vi "RainbowStationMain.vi"(8 "error in (no error)":errorcluster) -> (0 "error out":errorcluster={"status"=FALSE, "code"=1073676418, "source"="VISA Close in RainbowStationMain.vi"})   [LabVIEW 2013]
doc: "Use this template to build a VI to use as a subVI."
uses:
  GRIMM/GRIMMstatusEnum.ctl
  GRIMM/GRIMMmeasurementEnum.ctl
  HighVolumeSampler/HVSmeasurementEnum.ctl
  <vilib>/Instr/_visa.llb/Select Event Type.ctl
  Nephelometer/NephDataEnum.ctl
  GRIMM/GRIMMErrorMessage.ctl
  GRIMM/GRIMMmeasurementCluster.ctl
  <vilib>/Instr/_visa.llb/VISA Configure Serial Port (Instr).vi
  <vilib>/Utility/file.llb/Write To Spreadsheet File (string).vi
  HighVolumeSampler/X-Modem_Labview85/Xmodem VISA.llb/XMODEM Type.ctl
panel:
  out "Pressure (mbar)":dbl(slide)=1007.3810320000001 scale=1000.0..1020.0
  out "Wind Direction":i32(knob)=170 scale=0.0..359.0
  out "Wind Speed":dbl(knob)=0.014 scale=0.0..28.0
  out "Humidity":dbl(slide)=48.6 scale=0.0..100.0
  out "Temperature":dbl(slide)=20.789 scale=0.0..100.0
  in  "error in (no error) 3":errorcluster
  out "XY Graph":cluster{dbl[], dbl[]}[](graph)=[{[0.25, 0.28], [1170.3030084322447, 1170.3030084322447]}, {[0.28, 0.3], [1293.252048081437, 1293.252048081437]}, {[0.3, 0.35], [433.9267074685252, 433.9267074685252]}, {[0.35, 0.4], [288.83320655615836, 288.83320655615836]}, {[0.4, 0.45], [74.28763662454614, 74.28763662454614]}, {[0.45, 0.5], [40.43053885454822, 40.43053885454822]}, {[0.5, 0.58], [42.66344688970791, 42.66344688970791]}, {[0.58, 0.65], [14.145596928722288, 14.145596928722288]}, {[0.65, 0.7], [21.74947604493162, 21.74947604493162]}, {[0.7, 0.8], [14.65720749687968, 14.65720749687968]}, {[0.8, 1.0], [8.255080926812933, 8.255080926812933]}, {[1.0, 1.3], [2.632887254292233, 2.632887254292233]}, {[1.3, 1.6], [2.2178695214687925, 2.2178695214687925]}, {[1.6, 2.0], [3.09565534755485, 3.09565534755485]}, {[2.0, 2.5], [2.373335766458719, 2.373335766458719]}, {[2.5, 3.0], [1.010340250921067, 1.010340250921067]}, {[3.0, 3.5], [1.1949788845949056, 1.1949788845949056]}, {[3.5, 4.0], [0.8621886762870412, 0.8621886762870412]}, {[4.0, 5.0], [0.9286966042664552, 0.9286966042664552]}, {[5.0, 6.5], [0.08776290847640775, 0.08776290847640775]}, {[6.5, 7.5], [0.0, 0.0]}, {[7.5, 8.5], [0.0, 0.0]}, {[8.5, 10.0], [0.0, 0.0]}, {[10.0, 12.5], [0.1031885115851617, 0.1031885115851617]}, {[12.5, 15.0], [0.0, 0.0]}, {[15.0, 17.5], [0.0, 0.0]}, {[17.5, 20.0], [0.0, 0.0]}, {[20.0, 25.0], [0.0, 0.0]}, {[25.0, 30.0], [0.0, 0.0]}, {[30.0, 32.0], [0.0, 0.0]}]
  out "Number of Particles":i32[](array[numeric])=[15495, 9735, 5860, 2955, 1280, 900, 715, 440, 370, 300, 215, 135, 105, 85, 55, 32, 32, 24, 16, 11, 2, 1, 1, 1, 1, 0, 0, 0, 0, 0, 0, 0]
  in  "error in (no error) 2":errorcluster
  in  "Save HVS file":bool
  in  "HVS File Path":path
  in  "HVS Com Port":refnum<visa-resource-name>="COM1"
  in  "Simulation Mode":bool
  in  "Set Interval Time Button":bool
  in  "Interval Time":T1(ring)=enum."6 Seconds"
  in  "Stop GRIMM Measurement":bool
  in  "Start GRIMM Measurement":bool
  in  "stop":bool
  in  "Save GRIMM file":bool
  in  "GRIMM File Path":path
  in  "GRIMM Com Port":refnum<visa-resource-name>="COM2"
  in  "Save Neph File":bool
  in  "File Path Control":path=path "T:/LabBox/Software/Airphoton Nephelometer/TestMean.csv"
  in  "Nephelometer Com Port":refnum<visa-resource-name>="COM17"
  out "Total Scattering (Red (632nm), Green (532nm), Blue (450nm))":waveform(dbl)[](graph)=[{"t0"=timestamp(3528791463.22 s since 1904-01-01), "dt"=1.0, "Y"=[11.768620561478]}, {"t0"=timestamp(3528791463.22 s since 1904-01-01), "dt"=1.0, "Y"=[10.3616270811]}, {"t0"=timestamp(3528791463.22 s since 1904-01-01), "dt"=1.0, "Y"=[32.318224076812]}]
  out "External Sensors":waveform(dbl)[](graph)=[{"t0"=timestamp(3528791463.22 s since 1904-01-01), "dt"=1.0, "Y"=[24.22]}, {"t0"=timestamp(3528791463.22 s since 1904-01-01), "dt"=1.0, "Y"=[101.15]}, {"t0"=timestamp(3528791463.22 s since 1904-01-01), "dt"=1.0, "Y"=[48.6]}]
  out "Counts vs Time":waveform(dbl)[](graph)=[{"t0"=timestamp(3528791463.266 s since 1904-01-01), "dt"=1.0, "Y"=[154.95000000000002]}, {"t0"=timestamp(3528791463.266 s since 1904-01-01), "dt"=1.0, "Y"=[153.60000000000002]}, {"t0"=timestamp(3528791463.266 s since 1904-01-01), "dt"=1.0, "Y"=[154.63000000000002]}, {"t0"=timestamp(3528791463.266 s since 1904-01-01), "dt"=1.0, "Y"=[154.94000000000003]}]
  out "Meterological Data":waveform(dbl)[](graph)=[{"t0"=timestamp(3528791462.555 s since 1904-01-01), "dt"=1.0, "Y"=[755.6]}, {"t0"=timestamp(3528791462.555 s since 1904-01-01), "dt"=1.0, "Y"=[20.789]}]
  out "Meterological Data 2":waveform(dbl)[](graph)=[{"t0"=timestamp(3528791462.555 s since 1904-01-01), "dt"=1.0, "Y"=[0.014]}, {"t0"=timestamp(3528791462.555 s since 1904-01-01), "dt"=1.0, "Y"=[169.94]}]
  out "High Volume Sampler - Sampling Data":waveform(dbl)[](graph)=[{"t0"=timestamp(3528791462.555 s since 1904-01-01), "dt"=1.0, "Y"=[0.0]}, {"t0"=timestamp(3528791462.555 s since 1904-01-01), "dt"=1.0, "Y"=[0.0]}, {"t0"=timestamp(3528791462.555 s since 1904-01-01), "dt"=1.0, "Y"=[0.0]}]
  out "XY Graph 2":cluster{dbl[], dbl[]}[](graph)=[{[0.25, 0.28], [57.60000000000001, 57.60000000000001]}, {[0.28, 0.3], [38.75000000000001, 38.75000000000001]}, {[0.3, 0.35], [29.05, 29.05]}, {[0.35, 0.4], [16.75, 16.75]}, {[0.4, 0.45], [3.8000000000000007, 3.8000000000000007]}, {[0.45, 0.5], [1.8499999999999996, 1.8499999999999996]}, {[0.5, 0.58], [2.75, 2.75]}, {[0.58, 0.65], [0.7000000000000002, 0.7000000000000002]}, {[0.65, 0.7], [0.7000000000000002, 0.7000000000000002]}, {[0.7, 0.8], [0.8500000000000001, 0.8500000000000001]}, {[0.8, 1.0], [0.7999999999999998, 0.7999999999999998]}, {[1.0, 1.3], [0.30000000000000004, 0.30000000000000004]}, {[1.3, 1.6], [0.20000000000000007, 0.20000000000000007]}, {[1.6, 2.0], [0.29999999999999993, 0.29999999999999993]}, {[2.0, 2.5], [0.23000000000000004, 0.23000000000000004]}, {[2.5, 3.0], [0.08000000000000002, 0.08000000000000002]}, {[3.0, 3.5], [0.07999999999999999, 0.07999999999999999]}, {[3.5, 4.0], [0.05, 0.05]}, {[4.0, 5.0], [0.09, 0.09]}, {[5.0, 6.5], [0.01, 0.01]}, {[6.5, 7.5], [0.0, 0.0]}, {[7.5, 8.5], [0.0, 0.0]}, {[8.5, 10.0], [0.0, 0.0]}, {[10.0, 12.5], [0.01, 0.01]}, {[12.5, 15.0], [0.0, 0.0]}, {[15.0, 17.5], [0.0, 0.0]}, {[17.5, 20.0], [0.0, 0.0]}, {[20.0, 25.0], [0.0, 0.0]}, {[25.0, 30.0], [0.0, 0.0]}, {[30.0, 32.0], [0.0, 0.0]}]
  out "Battery Power (%)":i32
  out "Power Supply Type":T2(ring)
  out "Pump Current (%)":i32 format="Pump Current %.0f %%"
  out "Error Messages":u16(ring) items=["New SELF-TEST: Fault Self-Test"=128, "No Memory Card"=64, "Check Nozzle: Whirls > 5%"=32, "No Operation: Battery Capacity = 0%"=16, "Please Recharge: Battery Capacity < 10%"=8, "Pump Current too High - Motor Current Imot > 100%"=4, "Flow-Error: Volume flow control out of control range"=3, "Check Filter Imot < 20% "=2, "Check Filter Imot > 60%"=1, "No Error :)"=0]
  out "read buffer 2":string="1024,9/17/15 10:52:54,3093186,10310875,2353742,4299422,4381491,6981848,1595346,20761660,1351020,7590174,2065561,14187844,24.22,101.15,48.6,874857,984521,1006387,4.775941096085,5.786920205497,5.869425532089,11.768620561478,10.361627081100,32.318224076812,0\u0000"
  out "read buffer":string="C9:   15495     9735     5860     2955     1280      900      715      440 \nC9;     370      300      215      135      105       85       55       32 \nc9:      32       24       16       11        2        1        1        1 \nc9;       1        0        0        0        0        0        0        0 \n"
  in  "error in (no error) 5":errorcluster
  out "HVS RAW data":string
  in  "Array":dbl[](array[numeric])
  out "error out 2":errorcluster
  in  "error in (no error) 4":errorcluster
  # "m/s"
  # "%"
  # "C"
  # "N"
  # "W"
  # "E"
  # "S"
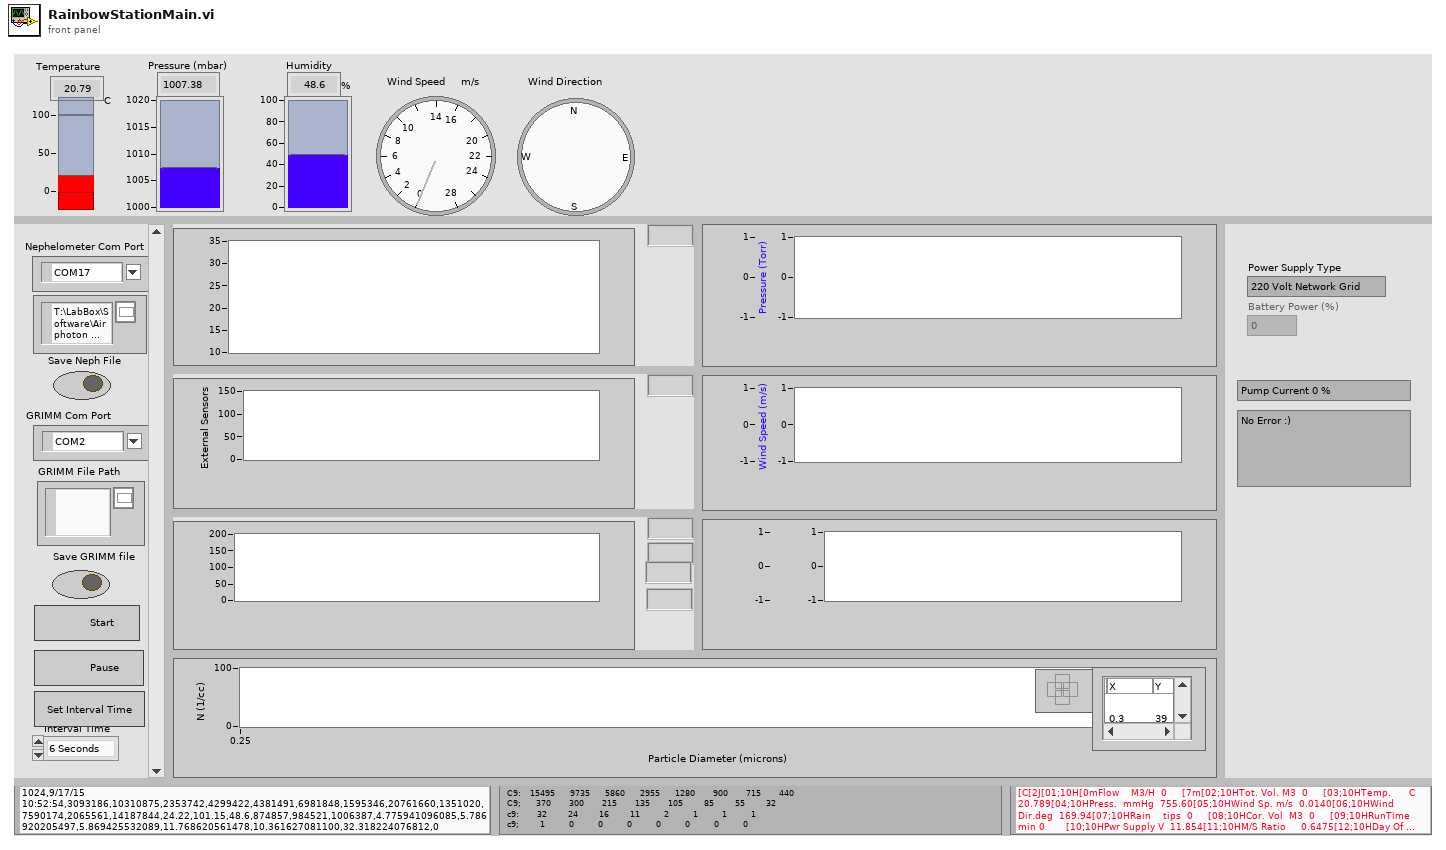
[diagram p1: front panel]
types:
  T1 = enum16{"1 Minute", "5 Mintues", "10 Minutes", "15 Minutes", "30 Minutes", "60 Minutes", "6 Seconds", "3 Seconds", "2 Seconds", "1 Second"}
  T2 = enum16{"220 Volt Network Grid", "Battery Powered"}
  T3 = typedef "NephDataEnum.ctl" = enum16{"Init", "Insert Measurement", "Read Buffer Size", "Write Buffer Size", "Read Current Measurement", "Read All Buffered Meas"}
  T4 = typedef "Select Event Type.ctl" = u32
  T5 = typedef "HVSmeasurementEnum.ctl" = enum16{"Get WindSpeedDirectionVsTime", "Get VolumeFlowrateVsTime", "Get PressureTempVsTime", "InsertMeasurement", "Init"}
  T6 = typedef "GRIMMmeasurementEnum.ctl" = enum16{"Save Raw to file", "Get NvsDiameter", "Get DNDlogDPVsDiameter", "Get CountsVsTime", "Get Raw Data", "InsertMeasurement", "Init"}
  T7 = typedef "GRIMMstatusEnum.ctl" = enum16{"Get Pump Current", "Get Power Supply Type", "Get Battery Power", "Get Error message", "Get Instrument DateTime", "Insert Status Data", "Init"}
  T8 = typedef "GRIMMmeasurementCluster.ctl" = cluster{"Threshold Bin size":dbl[], "Measurement Data":i32[]}
  T9 = enum8{"Enabled", "Disabled", "Disabled and Grayed Out"}
  T10 = typedef "GRIMMErrorMessage.ctl" = u16
  T11 = typedef "XMODEM Type.ctl" = enum16{"XMODEM", "XMODEM-CRC", "XMODEM-1K"}
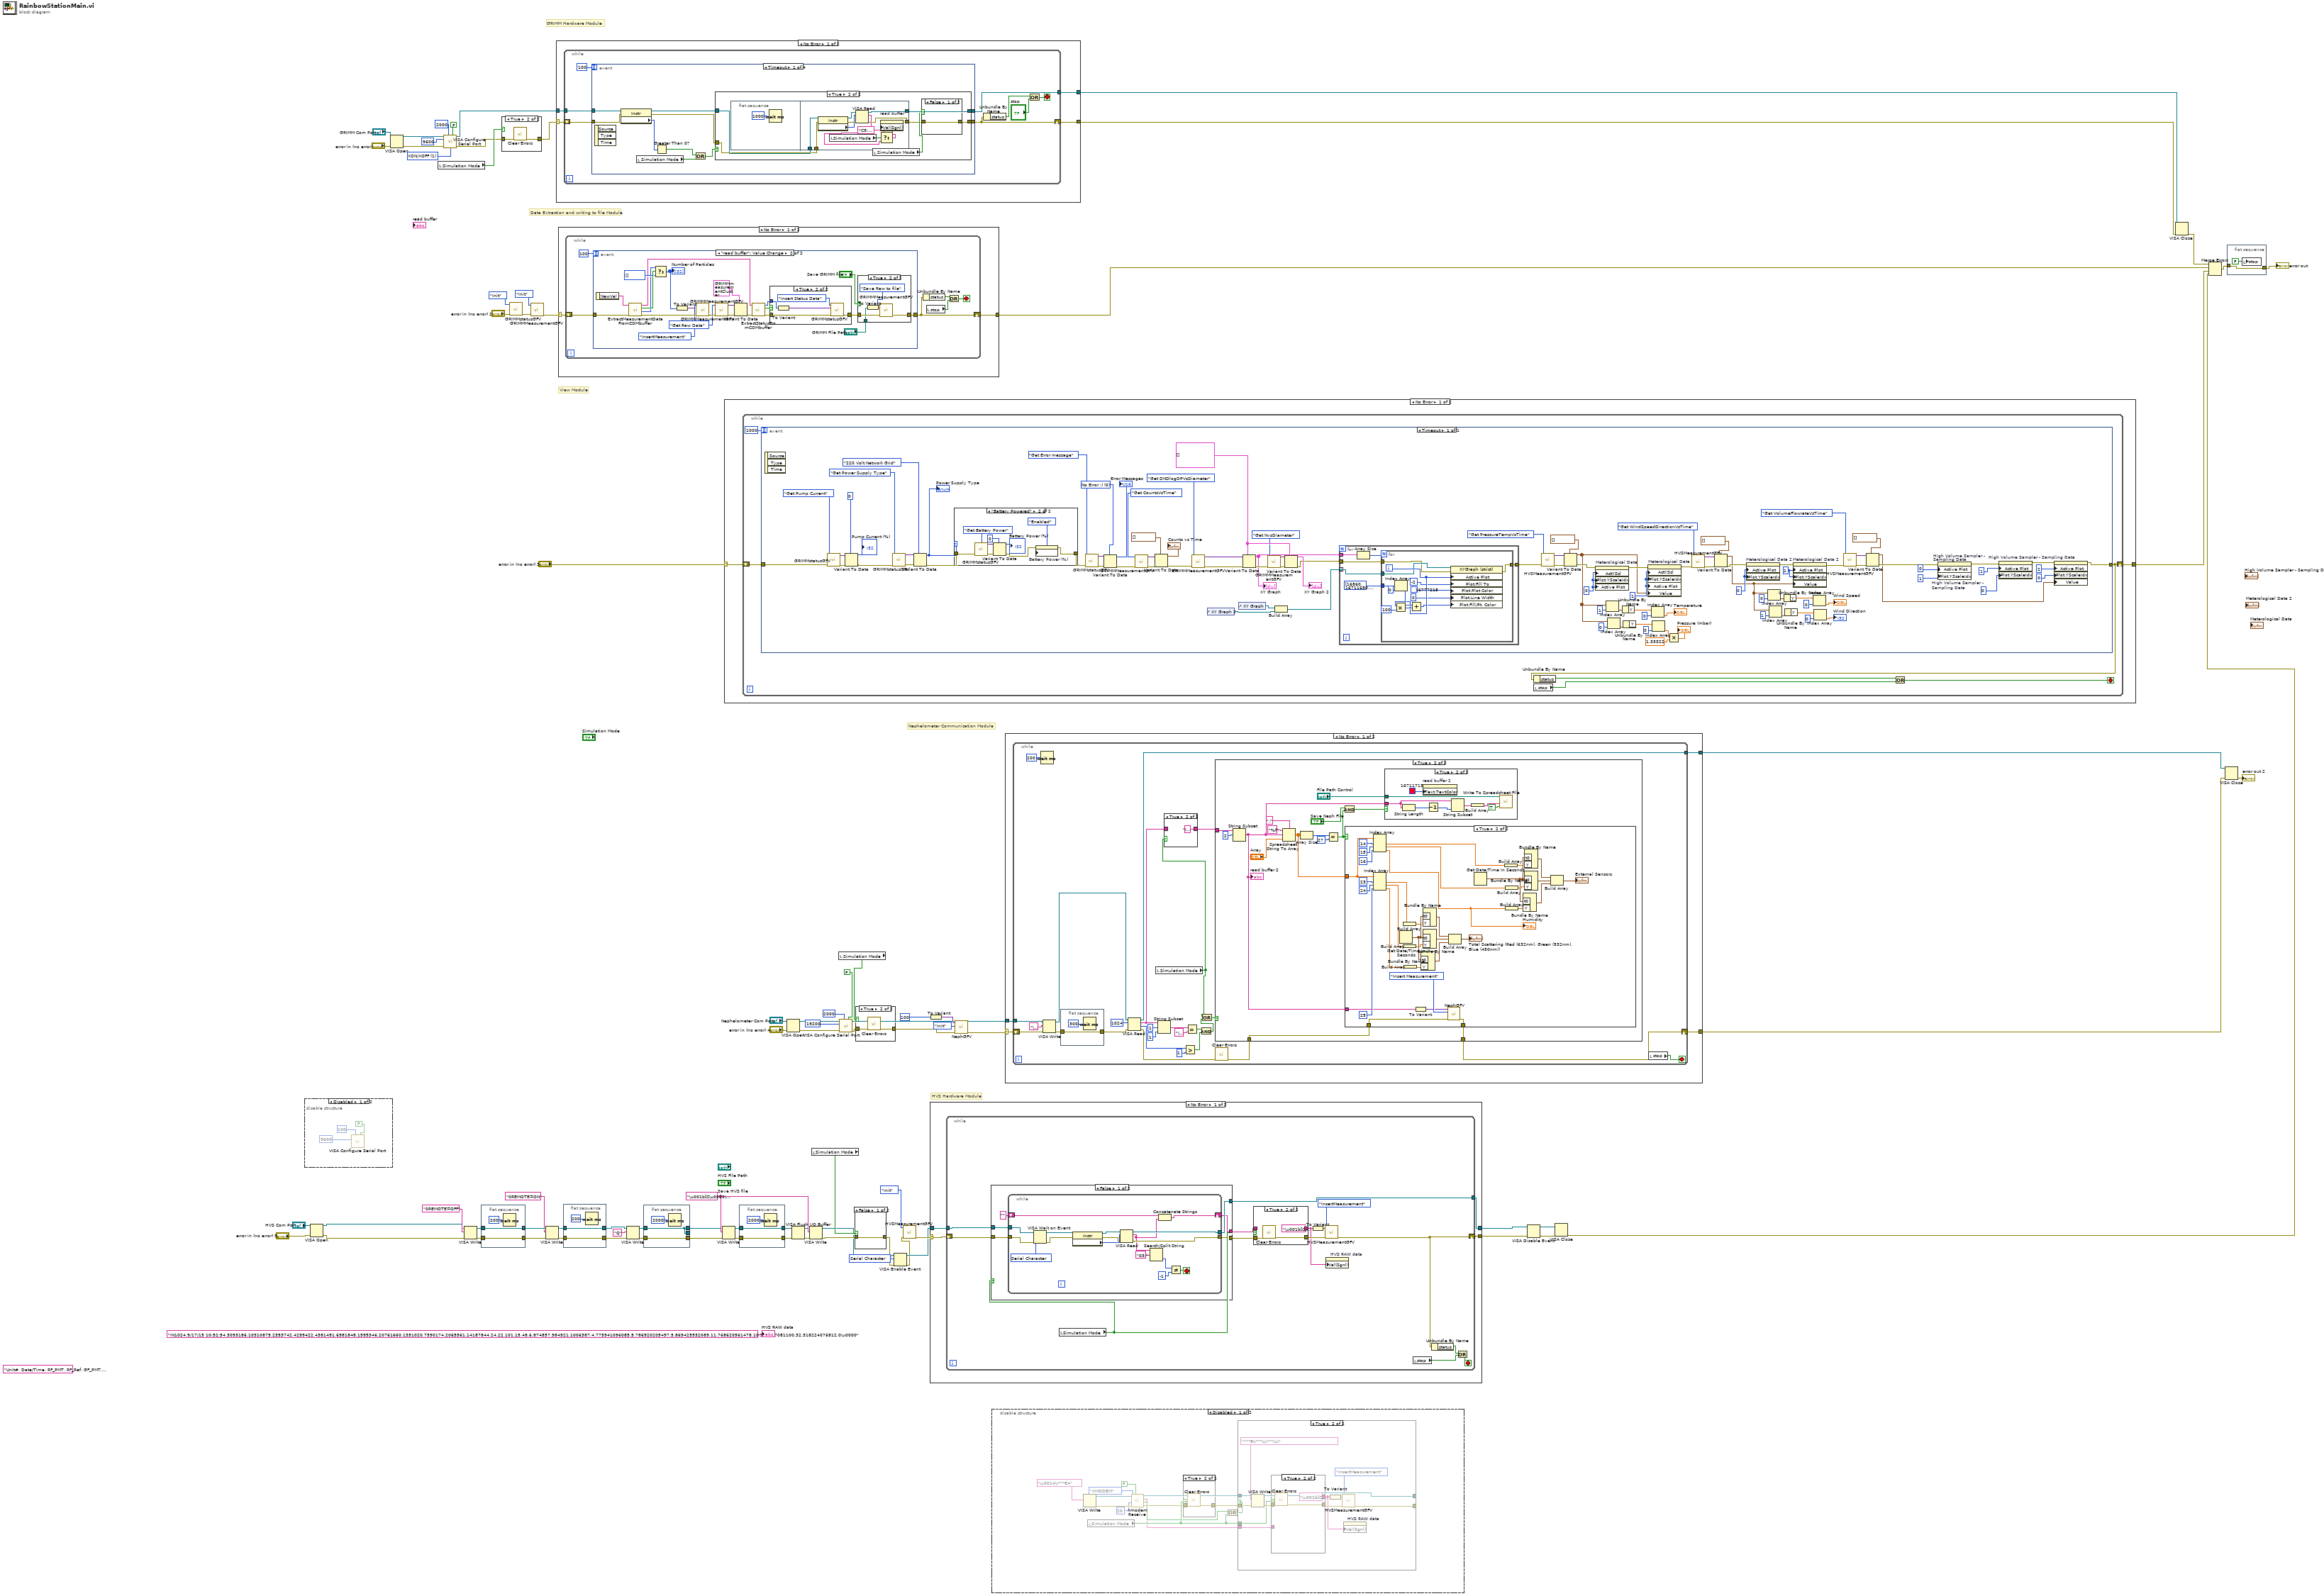
[diagram p0: block diagram]
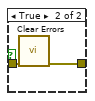
[diagram p7: hidden frame]
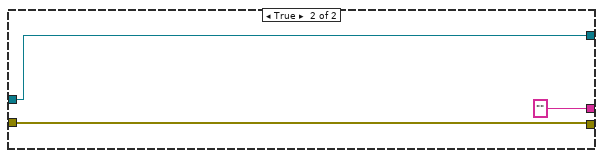
[diagram p8: hidden frame]
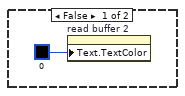
[diagram p16: hidden frame]
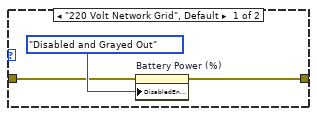
[diagram p18: hidden frame]
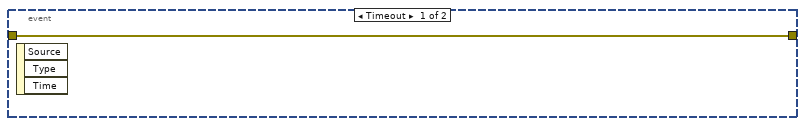
[diagram p20: hidden frame]
diagram:
  w6 = T4 1073684533 items=["Service Request"=1073684491, "Trigger"=3221168138, "Clear"=1073684493, "VXI Signal"=1073684512, "VXI/VME Interrupt"=3221168161, "VXI/VME Sysfail"=1073684509, "VXI/VME Sysreset"=1073684510, "GPIB CIC"=1073684498, "GPIB Talk"=1073684499, "GPIB Listen"=1073684500, "PXI Interrupt"=1073684514, "Serial Break"=1073684515, "Serial TermChar"=1073684516, "Serial CTS"=1073684521, "Serial DSR"=1073684522, "Serial DCD"=1073684524, "Serial RI"=1073684526, "Serial Character"=1073684533, "USB Interrupt"=1073684535, "All Enabled"=1073709055] ("Event Type")
  w39 = "\u001b[C\u0000\u0000" ("write buffer")
  (unwired) "Unit#, Date/Time, RF_PMT, RF_Ref, GF_PMT, GF_REF, BF_PMT, BF_REF, RB_PMT, RB_REF, GB_PMT, GB_REF, BB_PMT, BB_REF,Temp ,Pressure, RH%,  PMT DARK, Forw Dark Ref, Back Dark Ref, Back scatt Red, Back scatt Green, Back scatt Blue , Total scatt Red, Total scatt Green, Total scatt Blue, Fan RPM" ("write buffer")
  w77 = u16 1 items=["None", "XON/XOFF", "RTS/CTS", "XON/XOFF & RTS/CTS", "DTR/DSR", "XON/XOFF & DTR/DSR"] ("flow control (0:none)")
  # "HVS Hardware Module"
  # "Nephelometer Communication Module"
  # "View Module"
  # "Data Extraction and writing to file Module"
  # "GRIMM Hardware Module"
  n1 = disable-structure shown="Disabled" {
    frame Disabled {
      n2 = call-poly "VISA Configure Serial Port"("timeout (10sec)"=u32 100, "Enable Termination\nChar (T)"=FALSE ("Enable Termination\nChar (T)"), "baud rate (9600)"=u32 9600) -> ("VISA resource name"=w89:refnum<visa-resource-name>, "error in (no error)"=w88:errorcluster)  [unwired: 9 in, 2 out]
    }
    frame Enabled {
    }
  }
  n3 = VISA Open(error in (no error)="error in (no error) 5", VISA resource name="HVS Com Port") -> (VISA resource name=w16:refnum<visa-resource-name>, error out=w15:errorcluster)  [unwired: 3 in]
  n4 = VISA Open(error in (no error)="error in (no error)", VISA resource name="GRIMM Com Port") -> (VISA resource name=w84:refnum<visa-resource-name>, error out=w83:errorcluster)  [unwired: 3 in]
  n5 = local read "Simulation Mode"() -> (w51:bool)
  n6 = call-poly "VISA Configure Serial Port"("VISA resource name"=w84, "timeout (10sec)"=u32 2000, "Enable Termination\nChar (T)"=FALSE ("Enable Termination\nChar (T)"), "baud rate (9600)"=u32 9600, "error in (no error)"=w83, "flow control (0:none)"=w77) -> ("VISA resource name out"=w75:refnum<visa-resource-name>, "error out"=w50:errorcluster)  [unwired: 8 in]
  n7 = VISA Write(VISA resource name=w16, write buffer="0REMOTE=OFF", error in (no error)=w15) -> (VISA resource name out=w23:refnum<visa-resource-name>, error out=w21:errorcluster)  [unwired: 1 out]
  n8 = flat-sequence {
    tunnel: w21 -> [w91]
    tunnel: [w91] -> w22
    tunnel: w23 -> [w90]
    tunnel: [w90] -> w24
    frame #0 {
      n9 = Wait (ms)(milliseconds to wait=u32 200) -> ()  [unwired: 1 out]
    }
  }
  n10 = case shown="True" w51 {
    tunnel: w50 -> [w93 w95]
    tunnel: [w93 w94] -> w49
    frame False {
    }
    frame True {
      n11 = call <vilib>:"Clear Errors.vi"("error in (no error)"=w95) -> ("error out"=w94:errorcluster)  [unwired: 6 in]
    }
  }
  n12 = call "GRIMMstatusGFV.vi"("error in (no error)"="error in (no error) 2", "GrimmStatusEnum"=GRIMMstatusEnum."Init") -> ("error out"=w67:errorcluster)  [unwired: 8 in, 1 out]
  n13 = call "GRIMMMeasurementGFV.vi"("error in (no error)"=w67, "GRIMMMeasEnum"=GRIMMmeasurementEnum."Init") -> ("error out"=w65:errorcluster)  [unwired: 8 in, 1 out]
  n14 = VISA Write(VISA resource name=w24, write buffer="0REMOTE=ON", error in (no error)=w22) -> (VISA resource name out=w27:refnum<visa-resource-name>, error out=w25:errorcluster)  [unwired: 1 out]
  n15 = case shown="No Error" w49 {
    selector: w49 -> [w98 w180]
    tunnel: [w97 w180] -> w76
    tunnel: w75 -> [w99 w179]
    tunnel: [w96 w179] -> w74
    frame No Error {
      n16 = while {
        tunnel: w99 -> [w106]
        tunnel: [w105] -> w96
        shift-right: [w104] -> w97
        shift-left: w98 -> [w107]
        stop <- w101 stop-if-true
        n17 = event shown="[0] Timeout" {
          selector: _ -> [_ _ _ _]
          dyn-events: _ -> [_ _ _ _]
          timeout: 100 -> [_ _ _ _]
          tunnel: w107 -> [w114 w151 w171 w176]
          tunnel: [w108 w143 w170 w175] -> w104
          tunnel: [w112 w142 w169 w174] -> w105
          tunnel: w106 -> [w117 w150 w172 w177]
          event Timeout {
            n18 = event-data() -> ()  [unwired: 1 in, 3 out]
            n19 = property class="Instr"(reference=w117, error in=w114) -> (reference out=w115:refnum<visa-resource-name>, error out=w113:errorcluster, "Serial Settings:Number of Bytes at Serial Port"=w116:u32)
            n20 = local read "Simulation Mode"() -> (w111:bool)
            n21 = Greater Than 0?(x=w116) -> (x > 0?=w110:bool)
            n22 = Or(x=w110, y=w111) -> (x .or. y?=w109:bool)
            n23 = case shown="True" w109 {
              tunnel: w115 -> [w118 w125]
              tunnel: w113 -> [w119 w124]
              tunnel: [w118 w123] -> w112
              tunnel: [w119 w121] -> w108
              frame False {
              }
              frame True {
                n24 = flat-sequence {
                  tunnel: w125 -> [w140]
                  tunnel: w124 -> [w137]
                  tunnel: [w135] -> w123
                  tunnel: [w130] -> w120
                  frame #0 {
                    n25 = Wait (ms)(milliseconds to wait=u32 1000) -> ()  [unwired: 1 out]
                  }
                  frame #1 {
                    n26 = property class="Instr"(reference=w140, error in=w137) -> (reference out=w139:refnum<visa-resource-name>, error out=w136:errorcluster, "Serial Settings:Number of Bytes at Serial Port"=w138:u32)
                    n27 = local read "Simulation Mode"() -> (w134:bool)
                    n28 = VISA Read(VISA resource name=w139, byte count=w138, error in (no error)=w136) -> (VISA resource name out=w135:refnum<visa-resource-name>, read buffer=w133:string, error out=w130:errorcluster)  [unwired: 1 out]
                    n29 = Select(t="C9:   15495     9735     5860     2955     1280      900      715      440 \nC9;     370      300      215      135      105       85       55       32 \nc9:      32       24       16       11        2        1        1        1 \nc9;       1        0        0        0        0        0        0        0 \n", s=w134, f=w133) -> (s? t:f=w132:string)
                    n30 = property on="read buffer" class="Str"("Val(Sgnl)"=w132) -> ()  [unwired: 2 in, 2 out]
                  }
                }
                n31 = local read "Simulation Mode"() -> (w122:bool)
                n32 = case shown="False" w122 {
                  tunnel: w120 -> [w126 w128]
                  tunnel: [w126 w127] -> w121
                  frame False {
                  }
                  frame True {
                    n33 = call <vilib>:"Clear Errors.vi"("error in (no error)"=w128) -> ("error out"=w127:errorcluster)  [unwired: 6 in]
                  }
                }
              }
            }
          }
          event "Set Interval Time Button": Value Change {
            n34 = event-data() -> ()  [unwired: 1 in, 1 out]
            n35 = VISA Write(VISA resource name=w150, write buffer="I" ("string"), error in (no error)=w151) -> (VISA resource name out=w148:refnum<visa-resource-name>, error out=w147:errorcluster)  [unwired: 1 out]
            n36 = flat-sequence {
              tunnel: w148 -> [w153]
              tunnel: w147 -> [w152]
              tunnel: [w153] -> w146
              tunnel: [w152] -> w141
              tunnel: w146 -> [w158]
              tunnel: [w157] -> w145
              tunnel: [w156] -> w144
              tunnel: w141 -> [w155]
              tunnel: w145 -> [w166]
              tunnel: w144 -> [w165]
              tunnel: [w164] -> w143
              tunnel: [w163] -> w142
              frame #0 {
                n37 = Wait (ms)(milliseconds to wait=u32 500) -> ()  [unwired: 1 out]
              }
              frame #1 {
                n38 = property class="Instr"(reference=w158, error in=w155) -> (reference out=w161:refnum<visa-resource-name>, error out=w159:errorcluster, "Serial Settings:Number of Bytes at Serial Port"=w160:u32)
                n39 = VISA Read(VISA resource name=w161, byte count=w160, error in (no error)=w159) -> (VISA resource name out=w157:refnum<visa-resource-name>, error out=w156:errorcluster)  [unwired: 2 out]
              }
              frame #2 {
                n40 = Number To Decimal String(number="Interval Time", width (-)=i16 1) -> (decimal integer string=w162:string)
                n41 = VISA Write(VISA resource name=w166, write buffer=w162, error in (no error)=w165) -> (VISA resource name out=w163:refnum<visa-resource-name>, error out=w164:errorcluster)  [unwired: 1 out]
              }
            }
          }
          event "Start GRIMM Measurement": Value Change {
            n42 = event-data() -> ()  [unwired: 1 in, 1 out]
            n43 = VISA Write(VISA resource name=w172, write buffer="R", error in (no error)=w171) -> (VISA resource name out=w169:refnum<visa-resource-name>, error out=w170:errorcluster)  [unwired: 1 out]
          }
          event "Stop GRIMM Measurement": Value Change {
            n44 = event-data() -> ()  [unwired: 1 in, 1 out]
            n45 = VISA Write(VISA resource name=w177, write buffer="S", error in (no error)=w176) -> (VISA resource name out=w174:refnum<visa-resource-name>, error out=w175:errorcluster)  [unwired: 1 out]
          }
        }
        n46 = Unbundle By Name(w104) -> ("status"=w103:bool)
        n47 = Or(x=w103, y="stop") -> (x .or. y?=w101:bool)
      }
    }
    frame Error {
    }
  }
  n48 = case shown="No Error" w65 {
    selector: w65 -> [w182 w225]
    tunnel: [w181 w225] -> w73
    frame No Error {
      n49 = while {
        shift-right: [w186] -> w181
        shift-left: w182 -> [w188]
        stop <- w183 stop-if-true
        n50 = event shown="[1] \"read buffer\": Value Change" {
          selector: _ -> [_ _]
          dyn-events: _ -> [_ _]
          timeout: 100 -> [_ _]
          tunnel: w188 -> [w189 w211]
          tunnel: [w189 w192] -> w186
          event Timeout {
            n51 = event-data() -> ()  [unwired: 1 in, 3 out]
          }
          event "read buffer": Value Change {
            n52 = event-data() -> ("NewVal"=w212:string)  [unwired: 1 in]
            n53 = call "ExtractMeasurementDataFromCOMbuffer.vi"("error in (no error)"=w211, "Input OPC data"=w212) -> ("error out"=w206:errorcluster, "Output Number of Particles per 100 CC"=w208:i32[], "Valid Data"=w210:bool, "Output OPC data"=w207:string)  [unwired: 6 in]
            n54 = Select(t=w208, s=w210, f=i32[] []) -> (s? t:f=w203:i32[])
            "Number of Particles" <- w203
            n55 = To Variant(anything=w203) -> (Variant=w204:variant)
            n56 = call "GRIMMMeasurementGFV.vi"("error in (no error)"=w206, "Variant in"=w204, "GRIMMMeasEnum"=GRIMMmeasurementEnum."InsertMeasurement") -> ("error out"=w202:errorcluster)  [unwired: 7 in, 1 out]
            n57 = call "GRIMMMeasurementGFV.vi"("error in (no error)"=w202, "GRIMMMeasEnum"=GRIMMmeasurementEnum."Get Raw Data") -> ("error out"=w196:errorcluster, "Variant out"=w198:variant)  [unwired: 8 in]
            n58 = Variant To Data(error in=w196, type=T8 {"Threshold Bin size"=[], "Measurement Data"=[0, 0, 0, 0, 0, 0, 0, 1, 1, 1, 1, 1, 1, 2, 2, 2, 2, 3, 4, 4, 5, 6, 8, 8, 10, 12, 15, 18, 20, 25, 30, 32]}, Variant=w198) -> (error out=w200:errorcluster)  [unwired: 1 out]
            n59 = call "ExtractStatusFromCOMbuffer.vi"("error in (no error)"=w200, "Input OPC data"=w207) -> ("error out"=w197:errorcluster, "Valid Data"=w195:bool, "GRIMM STATUS"=w194:i32[])  [unwired: 7 in]
            n60 = case shown="True" w195 {
              tunnel: w197 -> [w219 w224]
              tunnel: [w219 w223] -> w193
              tunnel: w194 -> [_ w220]
              frame False {
              }
              frame True {
                n61 = To Variant(anything=w220) -> (Variant=w221:variant)
                n62 = call "GRIMMstatusGFV.vi"("error in (no error)"=w224, "Variant in"=w221, "GrimmStatusEnum"=GRIMMstatusEnum."Insert Status Data") -> ("error out"=w223:errorcluster)  [unwired: 7 in, 1 out]
              }
            }
            n63 = case shown="True" "Save GRIMM file" {
              tunnel: w193 -> [w213 w218]
              tunnel: [w213 w217] -> w192
              tunnel: "GRIMM File Path" -> [_ w215]
              frame False {
              }
              frame True {
                n64 = To Variant(anything=w215) -> (Variant=w216:variant)
                n65 = call "GRIMMMeasurementGFV.vi"("error in (no error)"=w218, "Variant in"=w216, "GRIMMMeasEnum"=GRIMMmeasurementEnum."Save Raw to file") -> ("error out"=w217:errorcluster)  [unwired: 7 in, 1 out]
              }
            }
          }
        }
        n66 = Unbundle By Name(w186) -> ("status"=w185:bool)
        n67 = local read "stop"() -> (w184:bool)
        n68 = Or(x=w185, y=w184) -> (x .or. y?=w183:bool)
      }
    }
    frame Error {
    }
  }
  n69 = flat-sequence {
    tunnel: w25 -> [w227]
    tunnel: [w227] -> w26
    tunnel: w27 -> [w226]
    tunnel: [w226] -> w28
    frame #0 {
      n70 = Wait (ms)(milliseconds to wait=u32 200) -> ()  [unwired: 1 out]
    }
  }
  n71 = VISA Write(VISA resource name=w28, write buffer="Q", error in (no error)=w26) -> (VISA resource name out=w30:refnum<visa-resource-name>, error out=w29:errorcluster)  [unwired: 1 out]
  n72 = flat-sequence {
    tunnel: w29 -> [w230]
    tunnel: [w230] -> w32
    tunnel: w30 -> [w229]
    tunnel: [w229] -> _
    tunnel: [w229] -> w31
    frame #0 {
      n73 = Wait (ms)(milliseconds to wait=u32 2000) -> ()  [unwired: 1 out]
    }
  }
  n74 = VISA Write(VISA resource name=w31, write buffer=w39, error in (no error)=w32) -> (VISA resource name out=w34:refnum<visa-resource-name>, error out=w33:errorcluster)  [unwired: 1 out]
  n75 = case shown="No Error" "error in (no error) 3" {
    selector: "error in (no error) 3" -> [w233 w369]
    tunnel: [w232 w369] -> w63
    frame No Error {
      n76 = while {
        shift-right: [w234] -> w232
        shift-left: w233 -> [w236]
        stop <- w237 stop-if-true
        n77 = event shown="[0] Timeout" {
          selector: _ -> [_]
          dyn-events: _ -> [_]
          timeout: 1000 -> [_]
          tunnel: w236 -> [w299]
          tunnel: [w267] -> w234
          event Timeout {
            w277 = u32 1 ("Active Plot")
            w279 = u32 0 ("Active Plot")
            w281 = 1 ("Active Y Scale")
            w283 = 0 ("Active Y Scale")
            w333 = cluster{dbl[], dbl[]}[] []
            w315 = T10 0 items=["New SELF-TEST: Fault Self-Test"=128, "No Memory Card"=64, "Check Nozzle: Whirls > 5%"=32, "No Operation: Battery Capacity = 0%"=16, "Please Recharge: Battery Capacity < 10%"=8, "Pump Current too High - Motor Current Imot > 100%"=4, "Flow-Error: Volume flow control out of control range"=3, "Check Filter Imot < 20% "=2, "Check Filter Imot > 60%"=1, "No Error :)"=0] ("Error Messages")
            n78 = event-data() -> ()  [unwired: 1 in, 3 out]
            n79 = call "GRIMMstatusGFV.vi"("error in (no error)"=w299, "GrimmStatusEnum"=GRIMMstatusEnum."Get Pump Current") -> ("error out"=w301:errorcluster, "Variant out"=w302:variant)  [unwired: 8 in]
            n80 = Variant To Data(error in=w301, type=0 ("Pump Current %"), Variant=w302) -> (data=→"Pump Current (%)":i32, error out=w305:errorcluster)
            n81 = call "GRIMMstatusGFV.vi"("error in (no error)"=w305, "GrimmStatusEnum"=GRIMMstatusEnum."Get Power Supply Type") -> ("error out"=w307:errorcluster, "Variant out"=w308:variant)  [unwired: 8 in]
            n82 = Variant To Data(error in=w307, type=T2."220 Volt Network Grid" ("Power Supply"), Variant=w308) -> (data=w310:T2, error out=w311:errorcluster)
            "Power Supply Type" <- w310
            n83 = case shown="\"Battery Powered\"" w310 {
              tunnel: w311 -> [w358 w368]
              tunnel: [w357 w360] -> w312
              frame "220 Volt Network Grid", Default {
                n84 = property on="Battery Power (%)" class="DigNum (strict)"(error in=w358, "DisabledEnum"=T9."Disabled and Grayed Out" ("Disabled")) -> (error out=w357:errorcluster)  [unwired: 1 in, 1 out]
              }
              frame "Battery Powered" {
                n85 = call "GRIMMstatusGFV.vi"("error in (no error)"=w368, "GrimmStatusEnum"=GRIMMstatusEnum."Get Battery Power") -> ("error out"=w366:errorcluster, "Variant out"=w365:variant)  [unwired: 8 in]
                n86 = Variant To Data(error in=w366, type=0 ("Pump Current %"), Variant=w365) -> (data=→"Battery Power (%)":i32, error out=w362:errorcluster)
                n87 = property on="Battery Power (%)" class="DigNum (strict)"(error in=w362, "DisabledEnum"=T9."Enabled" ("Disabled")) -> (error out=w360:errorcluster)  [unwired: 1 in, 1 out]
              }
            }
            n88 = call "GRIMMstatusGFV.vi"("error in (no error)"=w312, "GrimmStatusEnum"=GRIMMstatusEnum."Get Error message") -> ("error out"=w314:errorcluster, "Variant out"=w317:variant)  [unwired: 8 in]
            n89 = Variant To Data(error in=w314, type=w315, Variant=w317) -> (data=→"Error Messages":T10, error out=w322:errorcluster)
            n90 = call "GRIMMMeasurementGFV.vi"("error in (no error)"=w322, "GRIMMMeasEnum"=GRIMMmeasurementEnum."Get CountsVsTime") -> ("error out"=w319:errorcluster, "Variant out"=w320:variant)  [unwired: 8 in]
            n91 = Variant To Data(error in=w319, type=waveform(dbl)[] [] ("appended array"), Variant=w320) -> (data=→"Counts vs Time":waveform(dbl)[], error out=w323:errorcluster)
            n92 = call "GRIMMMeasurementGFV.vi"("error in (no error)"=w323, "GRIMMMeasEnum"=GRIMMmeasurementEnum."Get DNDlogDPVsDiameter") -> ("error out"=w326:errorcluster, "Variant out"=w325:variant)  [unwired: 8 in]
            n93 = control-ref of="XY Graph 2"() -> (w336:refnum<vi>)
            n94 = control-ref of="XY Graph"() -> (w335:refnum<vi>)
            n95 = Variant To Data(error in=w326, type=w333, Variant=w325) -> (data=w327:cluster{dbl[], dbl[]}[], error out=w329:errorcluster)
            "XY Graph" <- w327
            n96 = call "GRIMMMeasurementGFV.vi"("error in (no error)"=w329, "GRIMMMeasEnum"=GRIMMmeasurementEnum."Get NvsDiameter") -> ("error out"=w331:errorcluster, "Variant out"=w332:variant)  [unwired: 8 in]
            n97 = Build Array(w335, w336) -> (w337:refnum<vi>[])
            n98 = Variant To Data(error in=w331, type=w333, Variant=w332) -> (data=→"XY Graph 2":cluster{dbl[], dbl[]}[], error out=w298:errorcluster)
            n99 = for {
              tunnel: [w342] -> w285
              tunnel: w327 -> [w341]
              tunnel: w337 -> [w339] mode=indexing
              tunnel: w298 -> [w338]
              n100 = Array Size(array=w341) -> (size(s)=w340:i32)
              n101 = for {
                N: w340 -> [_]
                tunnel: u32[] [16860, 16711680, 1175296, 16773632, 15679744, 16711925, 2818015, 4325415] -> [w356]
                tunnel: [w346] -> w342
                tunnel: w339 -> [w345]
                tunnel: w338 -> [w344]
                i -> [w351]
                n102 = Multiply(x=w351, y=100) -> (x*y=w353:i32)
                n103 = Index Array(array=w356, index=0) -> (element=w354:u32)
                n104 = Add(x=w354, y=w353) -> (x+y=w347:u32)
                n105 = property class="XYGraph (strict)"(reference=w345, error in=w344, "Active Plot"=w351, "Plot.Fill To"=i16 -2, "Plot.Plot Color"=u32 16777215, "Plot.Line Width"=u8 0, "Plot.Fill/Pt. Color"=w347) -> (error out=w346:errorcluster)  [unwired: 1 out]
              }
            }
            n106 = call "HVSMeasurementGFV.vi"("error in (no error)"=w285, "HVSenum"=HVSmeasurementEnum."Get PressureTempVsTime") -> ("error out"=w296:errorcluster, "Variant out"=w295:variant)  [unwired: 8 in]
            n107 = Variant To Data(error in=w296, type=waveform(dbl)[] [] ("appended array"), Variant=w295) -> (data=w244:waveform(dbl)[], error out=w284:errorcluster)
            n108 = property on="Meterological Data" class="WFChart (strict)"(error in=w284, "ActYScl"=w283, "Plot.YScaleIdx"=w283, "Active Plot"=w283) -> (error out=w282:errorcluster)  [unwired: 1 in, 1 out]
            n109 = Index Array(array=w244, index=1) -> (element=w246:waveform(dbl))
            n110 = Index Array(array=w244, index=0) -> (element=w252:waveform(dbl))
            n111 = Unbundle By Name(w246) -> ("Y"=w248:dbl[])
            n112 = Unbundle By Name(w252) -> ("Y"=w250:dbl[])
            n113 = property on="Meterological Data" class="WFChart (strict)"(error in=w282, "ActYScl"=w281, "Plot.YScaleIdx"=w281, "Active Plot"=w281, "Value"=w244) -> (error out=w280:errorcluster)  [unwired: 1 in, 1 out]
            n114 = Index Array(array=w248, index=0) -> (element=→"Temperature":dbl)
            n115 = Index Array(array=w250, index=0) -> (element=w241:dbl)
            n116 = Multiply(x=w241, y=1.33322 ("Humidity")) -> (x*y=→"Pressure (mbar)":dbl)
            n117 = call "HVSMeasurementGFV.vi"("error in (no error)"=w280, "HVSenum"=HVSmeasurementEnum."Get WindSpeedDirectionVsTime") -> ("error out"=w291:errorcluster, "Variant out"=w292:variant)  [unwired: 8 in]
            n118 = Variant To Data(error in=w291, type=waveform(dbl)[] [] ("appended array"), Variant=w292) -> (data=w258:waveform(dbl)[], error out=w276:errorcluster)
            n119 = property on="Meterological Data 2" class="WFChart (strict)"(error in=w276, "Active Plot"=w279, "Plot.YScaleIdx"=w279) -> (error out=w278:errorcluster)  [unwired: 1 in, 1 out]
            n120 = Index Array(array=w258, index=0) -> (element=w262:waveform(dbl))
            n121 = Index Array(array=w258, index=1) -> (element=w255:waveform(dbl))
            n122 = Unbundle By Name(w262) -> ("Y"=w260:dbl[])
            n123 = Unbundle By Name(w255) -> ("Y"=w257:dbl[])
            n124 = property on="Meterological Data 2" class="WFChart (strict)"(error in=w278, "Active Plot"=w277, "Plot.YScaleIdx"=w277, "Value"=w258) -> (error out=w275:errorcluster)  [unwired: 1 in, 1 out]
            n125 = Index Array(array=w260, index=0) -> (element=→"Wind Speed":dbl)
            n126 = Index Array(array=w257, index=0) -> (element=→"Wind Direction":dbl)
            n127 = call "HVSMeasurementGFV.vi"("error in (no error)"=w275, "HVSenum"=HVSmeasurementEnum."Get VolumeFlowrateVsTime") -> ("error out"=w289:errorcluster, "Variant out"=w288:variant)  [unwired: 8 in]
            n128 = Variant To Data(error in=w289, type=waveform(dbl)[] [] ("appended array"), Variant=w288) -> (data=w264:waveform(dbl)[], error out=w272:errorcluster)
            n129 = property on="High Volume Sampler - Sampling Data" class="WFChart (strict)"(error in=w272, "Active Plot"=u32 0 ("Plot.Y Scale Index"), "Plot.YScaleIdx"=u32 1 ("Plot.Y Scale Index")) -> (error out=w273:errorcluster)  [unwired: 1 in, 1 out]
            n130 = property on="High Volume Sampler - Sampling Data" class="WFChart (strict)"(error in=w273, "Active Plot"=u32 1 ("Plot.Y Scale Index"), "Plot.YScaleIdx"=u32 0 ("Plot.Y Scale Index")) -> (error out=w268:errorcluster)  [unwired: 1 in, 1 out]
            n131 = property on="High Volume Sampler - Sampling Data" class="WFChart (strict)"(error in=w268, "Active Plot"=u32 2 ("Plot.Y Scale Index"), "Plot.YScaleIdx"=u32 0 ("Plot.Y Scale Index"), "Value"=w264) -> (error out=w267:errorcluster)  [unwired: 1 in, 1 out]
          }
        }
        n132 = Unbundle By Name(w234) -> ("status"=w239:bool)
        n133 = local read "stop"() -> (w238:bool)
        n134 = Or(x=w239, y=w238) -> (x .or. y?=w237:bool)
      }
    }
    frame Error {
    }
  }
  n135 = flat-sequence {
    tunnel: w33 -> [w371]
    tunnel: [w371] -> w36
    tunnel: w34 -> [w370]
    tunnel: [w370] -> w35
    frame #0 {
      n136 = Wait (ms)(milliseconds to wait=u32 2000) -> ()  [unwired: 1 out]
    }
  }
  n137 = VISA Open(error in (no error)="error in (no error) 4", VISA resource name="Nephelometer Com Port") -> (VISA resource name=w57:refnum<visa-resource-name>, error out=w56:errorcluster)  [unwired: 3 in]
  n138 = VISA Flush I/O Buffer(VISA resource name=w35, error in (no error)=w36) -> (VISA resource name out=w37:refnum<visa-resource-name>, error out=w38:errorcluster)  [unwired: 1 in]
  n139 = VISA Write(VISA resource name=w37, write buffer=w39, error in (no error)=w38) -> (VISA resource name out=w10:refnum<visa-resource-name>, error out=w17:errorcluster)  [unwired: 1 out]
  n140 = local read "Simulation Mode"() -> (w46:bool)
  n141 = local read "Simulation Mode"() -> (w48:bool)
  n142 = call-poly "VISA Configure Serial Port"("VISA resource name"=w57, "timeout (10sec)"=u32 2000, "Enable Termination\nChar (T)"=FALSE ("Enable Termination\nChar (T)"), "baud rate (9600)"=u32 19200, "error in (no error)"=w56) -> ("VISA resource name out"=w59:refnum<visa-resource-name>, "error out"=w47:errorcluster)  [unwired: 9 in]
  n143 = case shown="False" w46 {
    tunnel: w17 -> [w373 w375]
    tunnel: [w373 w374] -> w8
    frame False {
    }
    frame True {
      n144 = call <vilib>:"Clear Errors.vi"("error in (no error)"=w375) -> ("error out"=w374:errorcluster)  [unwired: 6 in]
    }
  }
  n145 = case shown="True" w48 {
    tunnel: w47 -> [w376 w378]
    tunnel: [w376 w377] -> w5
    frame False {
    }
    frame True {
      n146 = call <vilib>:"Clear Errors.vi"("error in (no error)"=w378) -> ("error out"=w377:errorcluster)  [unwired: 6 in]
    }
  }
  n147 = VISA Enable Event(8:w8, 10:w6, 11:w10) -> (0:w7:errorcluster, 3:w9:refnum<visa-resource-name>)  [unwired: 1 in]
  n148 = call "HVSMeasurementGFV.vi"("error in (no error)"=w7, "HVSenum"=HVSmeasurementEnum."Init") -> ("error out"=w42:errorcluster)  [unwired: 8 in, 1 out]
  n149 = To Variant(anything=100) -> (Variant=w2:variant)
  n150 = case shown="No Error" w42 {
    selector: w42 -> [w381 w429]
    tunnel: [w382 w429] -> w14
    tunnel: w9 -> [w380 w428]
    tunnel: [w379 w428] -> w12
    frame No Error {
      n151 = while {
        shift-right: [w393] -> w382
        shift-left: w381 -> [w392]
        tunnel: w380 -> [w391]
        tunnel: [w390] -> w379
        stop <- w394 stop-if-true
        n152 = local read "Simulation Mode"() -> (w383:bool)
        n153 = case shown="False" w383 {
          tunnel: w391 -> [w401 w420]
          tunnel: w392 -> [w402 w422]
          tunnel: [w397 "" ("read buffer")] -> w385
          tunnel: [w400 w420] -> w390
          tunnel: [w399 w422] -> w384
          frame False {
            n154 = while {
              tunnel: [w418] -> w400
              tunnel: w401 -> [w407]
              tunnel: w402 -> [w406]
              tunnel: [w415] -> w399
              shift-right: [w408] -> w397
              shift-left: "" ("read buffer") -> [w410]
              stop <- w411 stop-if-true
              w403 = T4 1073684533 items=["Service Request"=1073684491, "Trigger"=3221168138, "Clear"=1073684493, "VXI Signal"=1073684512, "VXI/VME Interrupt"=3221168161, "VXI/VME Sysfail"=1073684509, "VXI/VME Sysreset"=1073684510, "GPIB CIC"=1073684498, "GPIB Talk"=1073684499, "GPIB Listen"=1073684500, "PXI Interrupt"=1073684514, "Serial Break"=1073684515, "Serial TermChar"=1073684516, "Serial CTS"=1073684521, "Serial DSR"=1073684522, "Serial DCD"=1073684524, "Serial RI"=1073684526, "Serial Character"=1073684533, "USB Interrupt"=1073684535, "All Enabled"=1073709055] ("Event Type")
              n155 = VISA Wait on Event(8:w406, 10:w403, 11:w407) -> (0:w404:errorcluster, 3:w405:refnum<visa-resource-name>)  [unwired: 2 in, 2 out]
              n156 = property class="Instr"(reference=w405, error in=w404) -> (reference out=w419:refnum<visa-resource-name>, error out=w416:errorcluster, "Serial Settings:Number of Bytes at Serial Port"=w417:u32)
              n157 = VISA Read(VISA resource name=w419, byte count=w417, error in (no error)=w416) -> (VISA resource name out=w418:refnum<visa-resource-name>, read buffer=w409:string, error out=w415:errorcluster)  [unwired: 1 out]
              n158 = Search/Split String(string=w409, search string/char (-)="03;") -> (offset of match=w412:i32)  [unwired: 1 in, 2 out]
              n159 = Concatenate Strings(w410, w409) -> (w408:string)
              n160 = Not Equal?(x=w412, y=-1 ("milliseconds to wait")) -> (x != y?=w411:bool)
            }
          }
          frame True {
          }
        }
        n161 = case shown="True" w383 {
          tunnel: [w423 w427] -> w387
          tunnel: [w424 "\u001b[C\u0000\u0000\u001b[2J\u001b[01;10H\u001b[0mFlow    M3/H  0     \u001b[7m\u001b[02;10HTot. Vol. M3  0     \u001b[03;10HTemp.      C  20.789\u001b[04;10HPress.  mmHg  755.60\u001b[05;10HWind Sp. m/s  0.0140\u001b[06;10HWind Dir.deg  169.94\u001b[07;10HRain    tips  0     \u001b[08;10HCor. Vol  M3  0     \u001b[09;10HRunTime min 0       \u001b[10;10HPwr Supply V  11.854\u001b[11;10HM/S Ratio     0.6475\u001b[12;10HDay Of Week   SUN   \u001b[13;10HStart Dt OK?  YES   \u001b[14;10HEnd Dt OK?    NO    \u001b[15;10HDayOWeek OK?  NO    \u001b[16;10HTime OK?      NO    \u001b[17;10HWind OK?      YES   \u001b[18;10HTrigger OK?   " ("Data Received")] -> w386
          tunnel: w385 -> [w424 _]
          tunnel: w384 -> [w423 w425]
          frame False {
          }
          frame True {
            n162 = call <vilib>:"Clear Errors.vi"("error in (no error)"=w425) -> ("error out"=w427:errorcluster)  [unwired: 6 in]
          }
        }
        n163 = To Variant(anything=w386) -> (Variant=w389:variant)
        n164 = call "HVSMeasurementGFV.vi"("error in (no error)"=w387, "Variant in"=w389, "HVSenum"=HVSmeasurementEnum."InsertMeasurement") -> ("error out"=w393:errorcluster)  [unwired: 7 in, 1 out]
        n165 = property on="HVS RAW data" class="Str"("Val(Sgnl)"=w386) -> ()  [unwired: 2 in, 2 out]
        n166 = local read "stop"() -> (w395:bool)
        n167 = Unbundle By Name(w393) -> ("status"=w396:bool)
        n168 = Or(x=w396, y=w395) -> (x .or. y?=w394:bool)
      }
    }
    frame Error {
    }
  }
  n169 = call "NephGFV.vi"("error in (no error)"=w5, "NephDataEnum"=NephDataEnum."Init", "Variant In"=w2) -> ("error out"=w4:errorcluster)  [unwired: 7 in, 1 out]
  n170 = disable-structure shown="Disabled" {
    frame Disabled {
      n171 = VISA Write(write buffer="\u0014\r***EA") -> (VISA resource name out=w434:refnum<visa-resource-name>, error out=w432:errorcluster)  [unwired: 2 in, 1 out]
      n172 = local read "Simulation Mode"() -> (w443:bool)
      n173 = call "Xmodem Receive.vi"("trim EOF"=FALSE, "error in (no error)"=w432, "Max Errors"=u32 20, "error checking"=XMODEM_Type."XMODEM", "port"=w434) -> ("error out"=w439:errorcluster, "Transfer Success"=w441:bool, "Data Received"=w438:string, "port"=w435:refnum<visa-resource-name>)  [unwired: 3 in]
      n174 = case shown="True" w443 {
        tunnel: w439 -> [w445 w447]
        tunnel: [w445 w446] -> w440
        frame False {
        }
        frame True {
          n175 = call <vilib>:"Clear Errors.vi"("error in (no error)"=w447) -> ("error out"=w446:errorcluster)  [unwired: 6 in]
        }
      }
      n176 = Or(x=w441, y=w443) -> (x .or. y?=w442:bool)
      n177 = case shown="True" w442 {
        tunnel: w440 -> [w449 w461]
        tunnel: w435 -> [w448 w460]
        tunnel: [w449 w457] -> w436
        tunnel: [w448 w458] -> w437
        tunnel: w438 -> [_ w451]
        tunnel: w443 -> [_ w452]
        frame False {
        }
        frame True {
          n178 = VISA Write(VISA resource name=w460, write buffer="***B\r***L\r***L\r", error in (no error)=w461) -> (VISA resource name out=w458:refnum<visa-resource-name>, error out=w454:errorcluster)  [unwired: 1 out]
          n179 = case shown="True" w452 {
            tunnel: w454 -> [w463 w466]
            tunnel: [w463 w465] -> w453
            tunnel: w451 -> [w462 _]
            tunnel: [w462 "\u001b[C\u0000\u0000\u001b[2J\u001b[01;10H\u001b[0mFlow    M3/H  0     \u001b[7m\u001b[02;10HTot. Vol. M3  0     \u001b[03;10HTemp.      C  20.789\u001b[04;10HPress.  mmHg  755.60\u001b[05;10HWind Sp. m/s  0.0140\u001b[06;10HWind Dir.deg  169.94\u001b[07;10HRain    tips  0     \u001b[08;10HCor. Vol  M3  0     \u001b[09;10HRunTime min 0       \u001b[10;10HPwr Supply V  11.854\u001b[11;10HM/S Ratio     0.6475\u001b[12;10HDay Of Week   SUN   \u001b[13;10HStart Dt OK?  YES   \u001b[14;10HEnd Dt OK?    NO    \u001b[15;10HDayOWeek OK?  NO    \u001b[16;10HTime OK?      NO    \u001b[17;10HWind OK?      YES   \u001b[18;10HTrigger OK?   " ("Data Received")] -> w450
            frame False {
            }
            frame True {
              n180 = call <vilib>:"Clear Errors.vi"("error in (no error)"=w466) -> ("error out"=w465:errorcluster)  [unwired: 6 in]
            }
          }
          n181 = To Variant(anything=w450) -> (Variant=w456:variant)
          n182 = call "HVSMeasurementGFV.vi"("error in (no error)"=w453, "Variant in"=w456, "HVSenum"=HVSmeasurementEnum."InsertMeasurement") -> ("error out"=w457:errorcluster)  [unwired: 7 in, 1 out]
          n183 = property on="HVS RAW data" class="Str"("Val(Sgnl)"=w450) -> ()  [unwired: 2 in, 2 out]
        }
      }
    }
    frame Enabled {
    }
  }
  n184 = case shown="No Error" w4 {
    selector: w4 -> [w469 w562]
    tunnel: [w468 w562] -> w61
    tunnel: [w467 w561] -> w62
    tunnel: w59 -> [w470 w561]
    frame No Error {
      n185 = while {
        tunnel: w470 -> [w496]
        shift-right: [w473] -> w468
        shift-left: w469 -> [w495]
        tunnel: [w490] -> w467
        stop <- w479 stop-if-true
        n186 = Wait (ms)(milliseconds to wait=u32 200) -> ()  [unwired: 1 out]
        n187 = VISA Write(VISA resource name=w496, write buffer="\u0005", error in (no error)=w495) -> (VISA resource name out=w494:refnum<visa-resource-name>, error out=w481:errorcluster)  [unwired: 1 out]
        n188 = flat-sequence {
          tunnel: w481 -> [w499]
          tunnel: [w499] -> w480
          frame #0 {
            n189 = Wait (ms)(milliseconds to wait=u32 300) -> ()  [unwired: 1 out]
          }
        }
        n190 = VISA Read(VISA resource name=w494, byte count=u32 1024, error in (no error)=w480) -> (VISA resource name out=w490:refnum<visa-resource-name>, read buffer=w475:string, return count=w489:u32, error out=w472:errorcluster)
        n191 = local read "Simulation Mode"() -> (w476:bool)
        n192 = String Subset(string=w475, offset (0)=1, length (rest)=1 ("length (rest)")) -> (substring=w486:string)
        n193 = case shown="True" w476 {
          tunnel: w475 -> [w497 _]
          tunnel: [w497 "IN1024,9/17/15 10:52:54,3093186,10310875,2353742,4299422,4381491,6981848,1595346,20761660,1351020,7590174,2065561,14187844,24.22,101.15,48.6,874857,984521,1006387,4.775941096085,5.786920205497,5.869425532089,11.768620561478,10.361627081100,32.318224076812,0\u0000" ("read buffer")] -> w474
          frame False {
          }
          frame True {
          }
        }
        n194 = Greater?(x=w489, y=u32 1) -> (0:w483:bool)
        n195 = Equal?(x=w486, y="\u0006" ("write buffer")) -> (x = y?=w484:bool)
        n196 = And(x=w484, y=w483) -> (x .and. y?=w478:bool)
        n197 = Or(x=w476, y=w478) -> (x .or. y?=w477:bool)
        n198 = call <vilib>:"Clear Errors.vi"("error in (no error)"=w472) -> ("error out"=w471:errorcluster)  [unwired: 6 in]
        n199 = case shown="True" w477 {
          tunnel: w474 -> [_ w516]
          tunnel: w471 -> [w501 w504]
          tunnel: [w501 w503] -> w473
          frame False {
          }
          frame True {
            n200 = String Subset(string=w516, offset (0)=2) -> (substring=w502:string)  [unwired: 1 in]
            "read buffer 2" <- w502
            n201 = Spreadsheet String To Array(delimiter (Tab)=",", format string="%f", spreadsheet string=w502, array type (2D Dbl)="Array") -> (array=w511:dbl[])
            n202 = Array Size(array=w511) -> (size(s)=w510:i32)
            n203 = Equal?(x=w510, y=27) -> (x = y?=w505:bool)
            n204 = And(x="Save Neph File", y=w505) -> (x .and. y?=w508:bool)
            n205 = case shown="True" w505 {
              tunnel: w511 -> [_ w545]
              tunnel: w504 -> [w517 w522]
              tunnel: [w517 w521] -> w503
              tunnel: w502 -> [_ w518]
              frame False {
              }
              frame True {
                n206 = Index Array(array=w545, index #1=14 ("index"), index #2=15 ("index"), index #3=16 ("index")) -> (element #1=w540:dbl, element #2=w539:dbl, element #3=w523:dbl)
                "Humidity" <- w523
                n207 = Index Array(array=w545, index #1=23 ("index"), index #2=24 ("index"), index #3=25 ("index")) -> (element #1=w530:dbl, element #2=w529:dbl, element #3=w528:dbl)
                n208 = Get Date/Time In Seconds() -> (seconds since 1Jan1904=w531:timestamp)
                n209 = Build Array(w530) -> (w525:dbl[])
                n210 = Build Array(w529) -> (w526:dbl[])
                n211 = Build Array(w528) -> (w527:dbl[])
                n212 = To Variant(anything=w518) -> (Variant=w519:variant)
                n213 = Bundle By Name("t0"=w531, "Y"=w527) -> (w532:waveform(dbl))  [unwired: 1 in]
                n214 = Bundle By Name("t0"=w531, "Y"=w525) -> (w534:waveform(dbl))  [unwired: 1 in]
                n215 = Bundle By Name("t0"=w531, "Y"=w526) -> (w533:waveform(dbl))  [unwired: 1 in]
                n216 = call "NephGFV.vi"("error in (no error)"=w522, "NephDataEnum"=NephDataEnum."Insert Measurement", "Variant In"=w519) -> ("error out"=w521:errorcluster)  [unwired: 7 in, 1 out]
                n217 = Build Array(w534, w533, w532) -> (→"Total Scattering (Red (632nm), Green (532nm), Blue (450nm))":waveform(dbl)[])
                n218 = Get Date/Time In Seconds() -> (seconds since 1Jan1904=w541:timestamp)
                n219 = Build Array(w540) -> (w538:dbl[])
                n220 = Build Array(w539) -> (w537:dbl[])
                n221 = Build Array(w523) -> (w536:dbl[])
                n222 = Bundle By Name("t0"=w541, "Y"=w536) -> (w542:waveform(dbl))  [unwired: 1 in]
                n223 = Bundle By Name("t0"=w541, "Y"=w538) -> (w544:waveform(dbl))  [unwired: 1 in]
                n224 = Bundle By Name("t0"=w541, "Y"=w537) -> (w543:waveform(dbl))  [unwired: 1 in]
                n225 = Build Array(w544, w543, w542) -> (→"External Sensors":waveform(dbl)[])
              }
            }
            n226 = case shown="True" w508 {
              tunnel: w502 -> [_ w555]
              tunnel: "File Path Control" -> [_ w554]
              frame False {
                n227 = property on="read buffer 2" class="Str"("Text.TextColor"=u32 0) -> ()  [unwired: 2 in, 2 out]
              }
              frame True {
                n228 = String Length(string=w555) -> (length=w559:i32)
                n229 = property on="read buffer 2" class="Str"("Text.TextColor"=u32 16711713) -> ()  [unwired: 2 in, 2 out]
                n230 = Decrement(x=w559) -> (x-1=w558:i32)
                n231 = String Subset(string=w555, length (rest)=w558) -> (substring=w557:string)  [unwired: 1 in]
                n232 = Build Array(w557) -> (w556:string[])
                n233 = call-poly <vilib>:"Write To Spreadsheet File.vi"("append to file? (new file:F)"=TRUE, "1D data"=w556, "file path (dialog if empty)"=w554) -> ()  [unwired: 5 in, 1 out]
              }
            }
          }
        }
        n234 = local read "stop"() -> (w479:bool)
      }
    }
    frame Error {
    }
  }
  n235 = VISA Disable Event(8:w14, 11:w12) -> (0:w13:errorcluster, 3:w11:refnum<visa-resource-name>)  [unwired: 2 in]
  n236 = VISA Close(VISA resource name=w11, error in (no error)=w13) -> (error out=w43:errorcluster)
  n237 = VISA Close(VISA resource name=w74, error in (no error)=w76) -> (error out=w72:errorcluster)
  n238 = Merge Errors(w72, w73, w63, w43) -> (w71:errorcluster)
  n239 = VISA Close(VISA resource name=w62, error in (no error)=w61) -> (error out=→"error out 2":errorcluster)
  n240 = flat-sequence {
    tunnel: w71 -> [w563]
    tunnel: [w563] -> w70
    frame #0 {
      n241 = local write "stop"(FALSE ("stop")) -> ()
    }
  }
  "error out" <- w70
  "HVS RAW data" <- "IN1024,9/17/15 10:52:54,3093186,10310875,2353742,4299422,4381491,6981848,1595346,20761660,1351020,7590174,2065561,14187844,24.22,101.15,48.6,874857,984521,1006387,4.775941096085,5.786920205497,5.869425532089,11.768620561478,10.361627081100,32.318224076812,0\u0000" ("HVS RAW data")
